vi "PWMout wrapper.vi"(11 "PWM in":T1) -> (3 "Value":bool)   [LabVIEW 2013]
uses:
  Typedefs/PWM.ctl
  <vilib>/NI Veristand/FPGA/NI_VS FPGA Support.lvlib
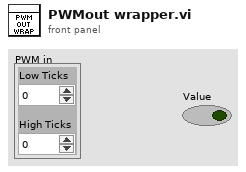
[diagram p1: front panel]
types:
  T1 = typedef "PWM.ctl" = cluster{"Low Ticks":u32, "High Ticks":u32}
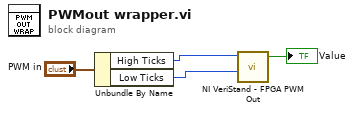
[diagram p0: block diagram]
diagram:
  n1 = Unbundle By Name("PWM in") -> ("High Ticks"=w2:u32, "Low Ticks"=w1:u32)
  n2 = call <vilib>:"NI VeriStand - FPGA PWM Out.vi"("_Low Time"=w1, "_High Time"=w2) -> ("Output"=→"Value":bool)  [unwired: 9 in]
